vi "sub_lidar_to_img.vi"(8 "error in":errorcluster) -> (0 "error out":errorcluster)   [LabVIEW 2019]
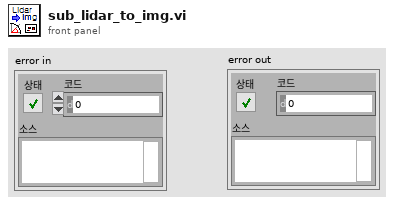
[diagram p1: front panel]
types:
  T1 = typedef "IMAQ Image.ctl" = refnum<image>
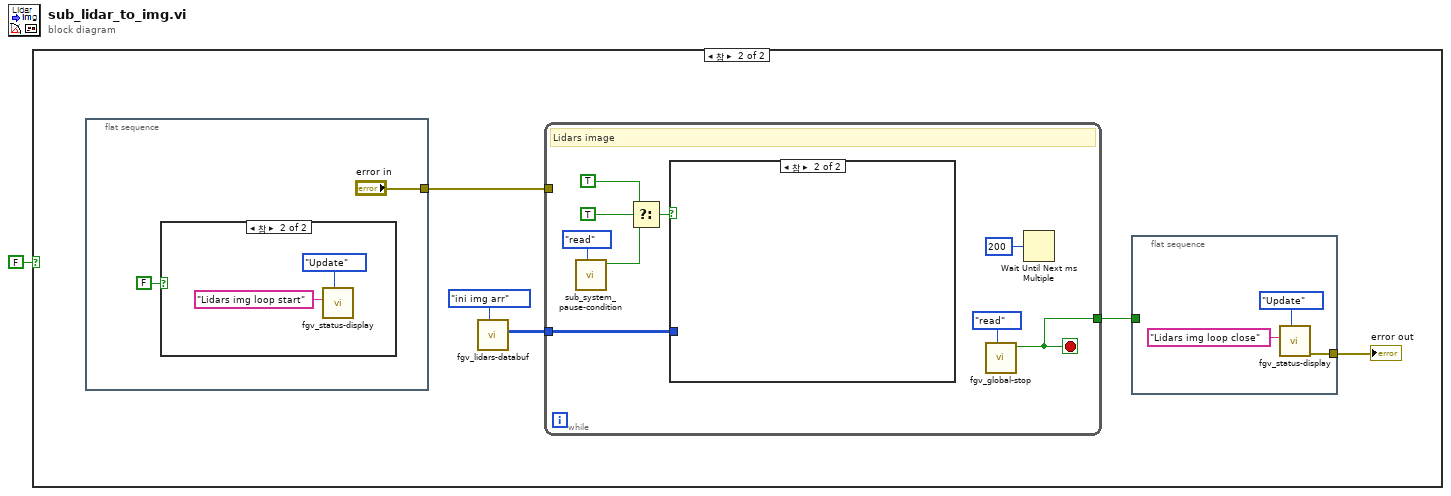
[diagram p0: block diagram]
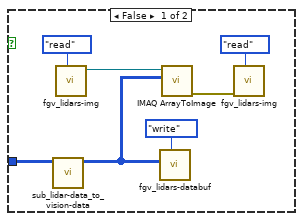
[diagram p4: hidden frame]
diagram:
  n1 = case shown="참" FALSE {
    frame False {
    }
    frame True {
      n2 = flat-sequence {
        tunnel: ["error in"] -> w2
        frame #0 {
          n3 = case shown="참" FALSE {
            frame False {
            }
            frame True {
              n4 = call "fgv_status-display.vi"("Mode"=enum16{"Initial", "Update", "Clear"}."Update", "title"="Lidars img loop start" ("String in 1")) -> ()  [unwired: 9 in, 1 out]
            }
          }
        }
      }
      n5 = call "fgv_lidars-databuf.vi"("cmd"=enum16{"ini img arr", "write", "read"}."ini img arr") -> ("img-data2d out"=w3:u8[][])  [unwired: 9 in, 1 out]
      n6 = while {
        tunnel: w3 -> [w21]
        tunnel: [w19] -> w4
        tunnel: w2 -> [_]
        stop <- w19 stop-if-true
        # "Lidars image"
        n7 = call "sub_system_pause-condition.vi"("cmd"=enum16{"pause", "go", "read"}."read") -> ("pause"=w17:bool)  [unwired: 10 in]
        n8 = Select(t=TRUE, s=TRUE, f=w17) -> (s? t:f=w14:bool)
        n9 = case shown="참" w14 {
          tunnel: w21 -> [w23 _]
          frame False {
            n10 = call "sub_lidar-data_to_vision-data.vi"("img-data2d in"=w23) -> ("img-data2d out"=w24:u8[][])  [unwired: 10 in]
            n11 = call "fgv_lidars-img.vi"("cmd"=enum16{"create", "read", "close"}."read") -> ("New Image"=w26:T1)  [unwired: 10 in]
            n12 = call "fgv_lidars-databuf.vi"("cmd"=enum16{"ini img arr", "write", "read"}."write", "img-data in"=w24) -> ()  [unwired: 8 in, 2 out]
            n13 = call "IMAQ ArrayToImage"("Image Pixels (U8)"=w24, "Image"=w26) -> ("error out"=w27:errorcluster)  [unwired: 8 in, 1 out]
            n14 = call "fgv_lidars-img.vi"("cmd"=enum16{"create", "read", "close"}."read", "error in (no error)"=w27) -> ()  [unwired: 9 in, 1 out]
          }
          frame True {
          }
        }
        n15 = call "fgv_global-stop.vi"("cmd"=enum16{"init", "stop", "read"}."read") -> ("val_out"=w19:bool)  [unwired: 10 in]
        n16 = Wait Until Next ms Multiple(millisecond multiple=u32 200) -> ()  [unwired: 1 out]
      }
      n17 = flat-sequence {
        tunnel: w4 -> [_]
        tunnel: [w11] -> w5
        frame #0 {
          n18 = call "fgv_status-display.vi"("Mode"=enum16{"Initial", "Update", "Clear"}."Update", "title"="Lidars img loop close" ("String in 1")) -> ("error out"=w11:errorcluster)  [unwired: 9 in]
        }
      }
      "error out" <- w5
    }
  }
